vi "CAN_enableOFF_individual.vi"(3 "Switch On":bool, 4 "Current":i32(slide) scale=-1000.0..1000.0, 5 "Array 3":errorcluster[](array[cluster]), 6 "Array 2":refnum<class "sbCANopenBaseClass.lvclass">[](array[class])) -> (0 "error out":errorcluster, 2 "CANopen Session Out":refnum<class "sbCANopenBaseClass.lvclass">)   [LabVIEW 2017]
uses:
  <vilib>/addons/Maxon Motor/EPOS2 CANopen/CANopen/sbCANopenBaseClass.lvclass
  <vilib>/addons/Maxon Motor/EPOS2 CANopen/EPOS2 Support Files/Typedefs/EPOS2 Control Word PVM.ctl
  <vilib>/addons/Maxon Motor/EPOS2 CANopen/EPOS2 Support Files/Polymorphic SubVIs/Write PDO/EPOS2 Current Mode Write.vi
  <vilib>/addons/Maxon Motor/EPOS2 CANopen/EPOS2 Support Files/Polymorphic SubVIs/Read PDO/EPOS2 Current Mode Read.vi
  <vilib>/addons/Maxon Motor/EPOS2 CANopen/EPOS2 Library.lvlib
panel:
  in  "index":i32
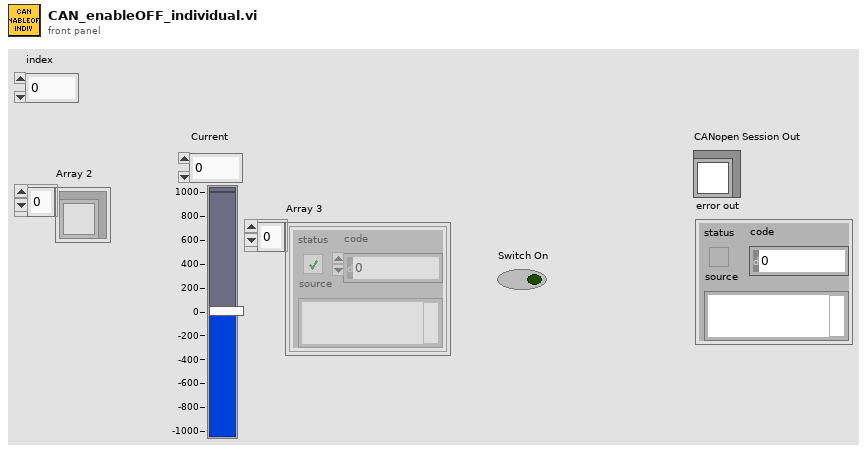
[diagram p1: front panel]
types:
  T1 = typedef "EPOS2 Library.lvlib/EPOS2 Control Word PVM.ctl" = cluster{"Switch On":bool, "Enable Voltage":bool, "Quick Stop":bool, "Enable Operation":bool, "Reserved 0":bool, "Reserved 1":bool, "Reserved 2":bool, "Fault Reset":bool, "Halt":bool}
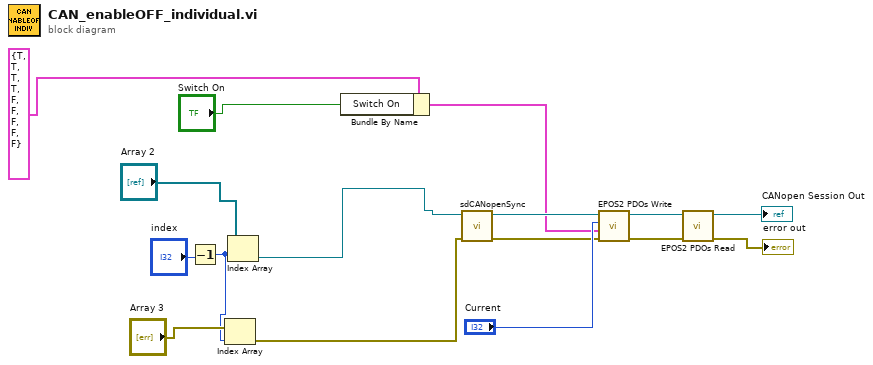
[diagram p0: block diagram]
diagram:
  n1 = Decrement(x="index") -> (x-1=w2:i32)
  n2 = Index Array(array="Array 3", index=w2) -> (element=w1:errorcluster)
  n3 = Index Array(array="Array 2", index=w2) -> (element=w5:refnum<class "sbCANopenBaseClass.lvclass">)
  n4 = Bundle By Name(cluster=T1 {"Switch On"=TRUE, "Enable Voltage"=TRUE, "Quick Stop"=TRUE, "Enable Operation"=TRUE, "Reserved 0"=FALSE, "Reserved 1"=FALSE, "Reserved 2"=FALSE, "Fault Reset"=FALSE, "Halt"=FALSE} ("Control Word"), "Switch On"="Switch On") -> (w12:T1)
  n5 = call-dynamic "sdCANopenSync.vi"("error in (no error)"=w1, "sbCANopenBaseClass in"=w5) -> ("error out"=w14:errorcluster, "sbCANopenBaseClass out"=w15:refnum<class "sbCANopenBaseClass.lvclass">)  [unwired: 8 in]
  n6 = call-poly <vilib>:"EPOS2 PDOs Write.vi"("error in"=w14, "Control Word"=w12, "Current"="Current", "CANopen Session In"=w15) -> ("error out"=w9:errorcluster, "CANopen Session Out"=w11:refnum<class "sbCANopenBaseClass.lvclass">)  [unwired: 6 in]
  n7 = call-poly <vilib>:"EPOS2 PDOs Read.vi"("error in"=w9, "CANopen Session In"=w11) -> ("error out"=→"error out":errorcluster, "CANopen Session Out"=→"CANopen Session Out":refnum<class "sbCANopenBaseClass.lvclass">)  [unwired: 6 in, 2 out]
